vi "Table.Clear.vi"(8 "error in (no error)":errorcluster, 11 "Cluster":T1) -> (0 "error out":errorcluster)   [LabVIEW 2015, in "Station.Execution.lvlib"]
uses:
  Station.Execution.lvlib
  Types/Main.StateVariables.ctl
  Types/Execute.UserEventRefs.ctl
  <vilib>/NI Veristand/Execution/Workspace/SystemStateRegEventRef.ctl
  <vilib>/NI Veristand/Execution/Workspace/Target State Info.ctl
  <vilib>/NI Veristand/Execution/Workspace/Target State.ctl
  <vilib>/NI Veristand/Execution/Workspace/SystemStateEventRef.ctl
  <vilib>/NI Veristand/Execution/Workspace/WorkspaceAPI.ctl
  NationalInstruments.VeriStand.ClientAPI
  Types/UI.Tables.ctl
  Types/UI.Object.ctl
  <vilib>/Utility/miscctls.llb/LVRowAndColumnTypeDef.ctl
  <vilib>/NI Veristand/Execution/Workspace/NI_VS Workspace ExecutionAPI.lvlib
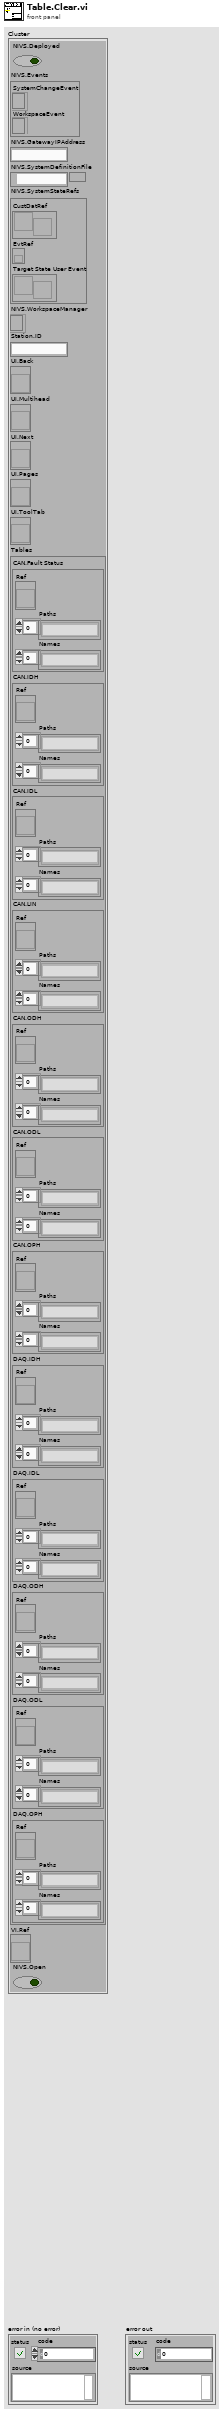
[diagram p1: front panel]
types:
  T1 = typedef "Station.Execution.lvlib/Main.StateVariables.ctl" = cluster{"NIVS.Deployed":bool, "NIVS.Events":T2, "NIVS.GatewayIPAddress":string, "NIVS.SystemDefinitionFile":path, "NIVS.SystemStateRefs":T4, "NIVS.WorkspaceManager":T5, "Station.ID":string, "UI.Back":refnum<vi>, "UI.Multihead":refnum<vi>, "UI.Next":refnum<vi>, "UI.Pages":refnum<vi>, "UI.ToolTab":refnum<vi>, "Tables":T6, "VI.Ref":refnum<vi>, "NIVS.Open":bool}
  T2 = typedef "Station.Execution.lvlib/Execute.UserEventRefs.ctl" = cluster{"SystemChangeEvent":T3, "WorkspaceEvent":refnum<event-registration>}
  T3 = typedef "NI_VS Workspace ExecutionAPI.lvlib/SystemStateRegEventRef.ctl" = refnum<event-registration>
  T4 = typedef "NI_VS Workspace ExecutionAPI.lvlib/SystemStateEventRef.ctl" = cluster{"CustDatRef":refnum<user-event>, "EvtRef":refnum<k27>, "Target State User Event":refnum<user-event>}
  T5 = typedef "NI_VS Workspace ExecutionAPI.lvlib/WorkspaceAPI.ctl" = refnum<k24>
  T6 = typedef "Station.Execution.lvlib/UI.Tables.ctl" = cluster{"CAN.Fault Status":T7, "CAN.IDH":T7, "CAN.IDL":T7, "CAN.LIN":T7, "CAN.ODH":T7, "CAN.ODL":T7, "CAN.OPH":T7, "DAQ.IDH":T7, "DAQ.IDL":T7, "DAQ.ODH":T7, "DAQ.ODL":T7, "DAQ.OPH":T7}
  T7 = typedef "Station.Execution.lvlib/UI.Object.ctl" = cluster{"Ref":refnum<vi>, "Paths":string[], "Names":string[]}
  T8 = typedef "LVRowAndColumnTypeDef.ctl" = cluster{"Row":i32, "Column":i32}
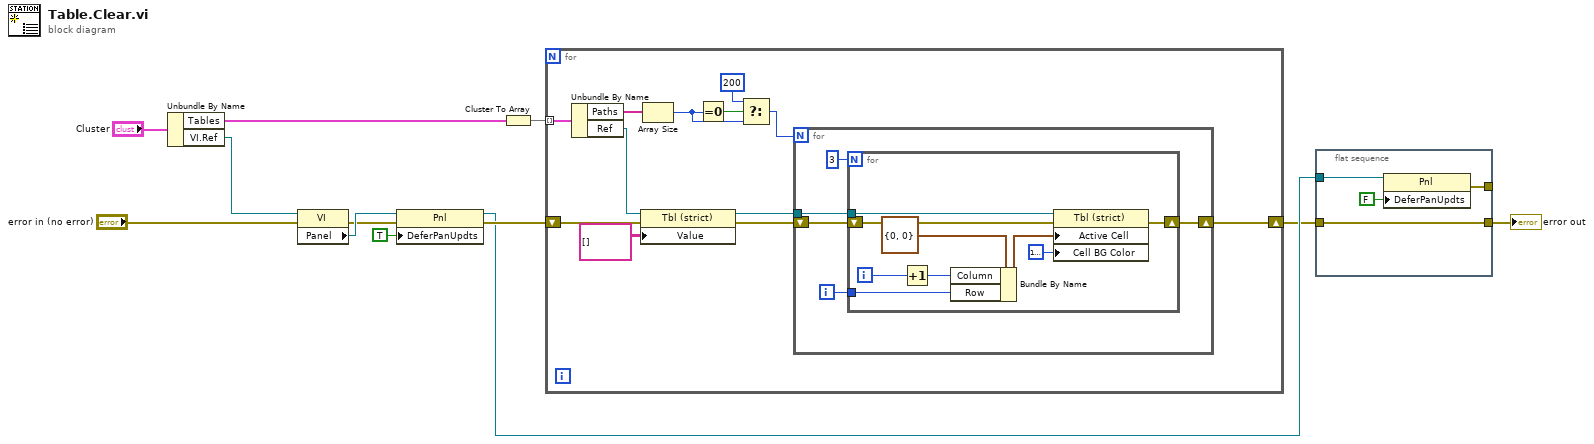
[diagram p0: block diagram]
diagram:
  n1 = Unbundle By Name("Cluster") -> ("Tables"=w11:T6, "VI.Ref"=w9:refnum<vi>)
  n2 = property class="VI"(reference=w9, error in="error in (no error)") -> (error out=w7:errorcluster, "Panel"=w8:refnum<vi>)  [unwired: 1 out]
  n3 = property class="Pnl"(reference=w8, error in=w7, "DeferPanUpdts"=TRUE ("Defer Panel Updates")) -> (reference out=w3:refnum<vi>, error out=w5:errorcluster)
  n4 = Cluster To Array(cluster=w11) -> (array=w10:T7[])
  n5 = for {
    shift-right: [w19] -> w1
    shift-left: w5 -> [w24]
    tunnel: w10 -> [w23] mode=indexing
    n6 = Unbundle By Name(w23) -> ("Paths"=w17:string[], "Ref"=w22:refnum<vi>)
    n7 = property class="Tbl (strict)"(reference=w22, error in=w24, "Value"=string[][] []) -> (reference out=w18:refnum<vi>, error out=w20:errorcluster)
    n8 = Array Size(array=w17) -> (size(s)=w14:i32)
    n9 = Equal To 0?(x=w14) -> (x = 0?=w16:bool)
    n10 = Select(t=200, s=w16, f=w14) -> (s? t:f=w13:i32)
    n11 = for {
      N: w13 -> [_]
      tunnel: w18 -> [w27]
      shift-right: [w28] -> w19
      shift-left: w20 -> [w29]
      i -> [w26]
      n12 = for {
        N: 3 -> [_]
        tunnel: w27 -> [w36]
        shift-right: [w37] -> w28
        shift-left: w29 -> [w38]
        tunnel: w26 -> [w30]
        i -> [w32]
        n13 = Increment(x=w32) -> (x+1=w31:i32)
        n14 = Bundle By Name(cluster=T8 {"Row"=0, "Column"=0} ("Active Cell:Active Cell"), "Column"=w31, "Row"=w30) -> (w33:T8)
        n15 = property class="Tbl (strict)"(reference=w36, error in=w38, "Active Cell"=w33, "Cell BG Color"=u32 16777216) -> (error out=w37:errorcluster)  [unwired: 1 out]
      }
    }
  }
  n16 = flat-sequence {
    tunnel: w3 -> [w42]
    tunnel: [w41] -> w2
    tunnel: w1 -> [w41]
    tunnel: [w40] -> _
    frame #0 {
      n17 = property class="Pnl"(reference=w42, "DeferPanUpdts"=FALSE ("Defer Panel Updates")) -> (error out=w40:errorcluster)  [unwired: 1 in, 1 out]
    }
  }
  "error out" <- w2
